vi "myPICO_ResultFFT.vi"(4 "是否需要第二台":bool, 5 "MultiBuffers 2":T1(array[cluster]), 6 "示波器量程":u16, 7 "MultiBuffers 1":T1(array[cluster]), 9 "Max Adc value 2":i16, 10 "Max Adc value":i16) -> (2 "数组":cdb[][](array[numeric]))   [LabVIEW 2024]
doc: "由于它的实际功能被合并进了myFFT_RowSave.vi\n（因为同步系模式需要在FFT前时域变换），\n实际上它并没有被在主程序中使用。"
uses:
  <vilib>/Analysis/2dsp.llb/Real FFT.vi
  <vilib>/Analysis/NI_AALPro.lvlib
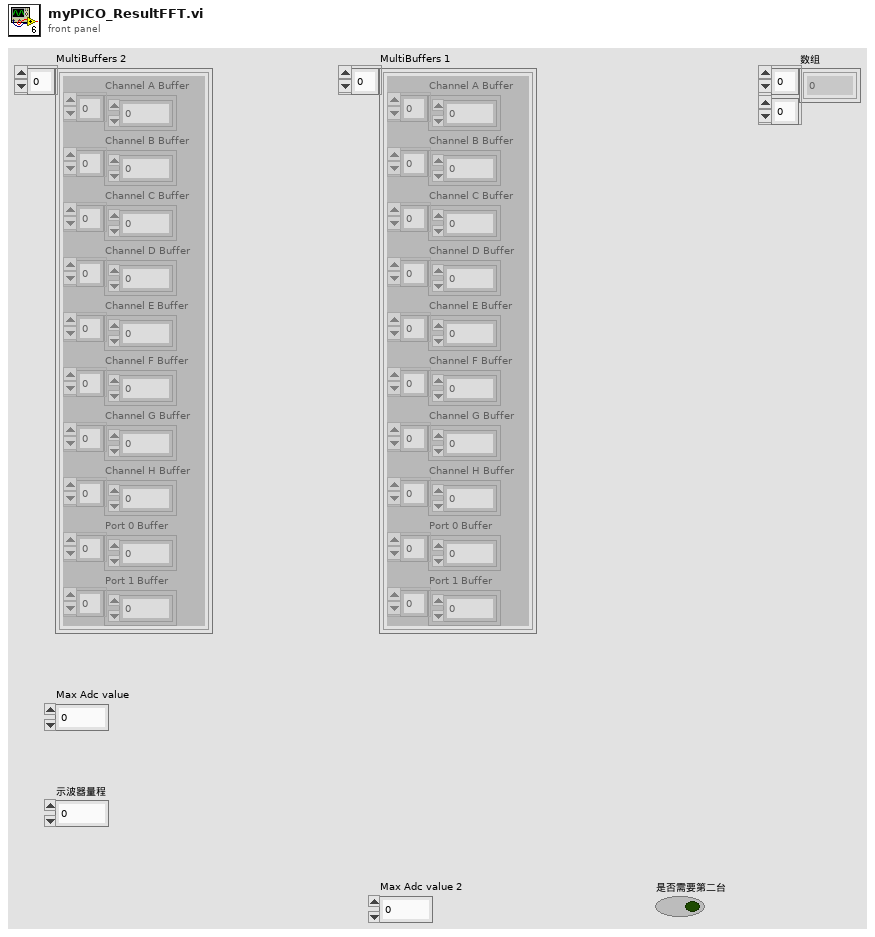
[diagram p1: front panel]
types:
  T1 = cluster{"Channel A Buffer":i16[], "Channel B Buffer":i16[], "Channel C Buffer":i16[], "Channel D Buffer":i16[], "Channel E Buffer":i16[], "Channel F Buffer":i16[], "Channel G Buffer":i16[], "Channel H Buffer":i16[], "Port 0 Buffer":i16[], "Port 1 Buffer":i16[]}[]
  T2 = cluster{"Channel A Buffer":i16[], "Channel B Buffer":i16[], "Channel C Buffer":i16[], "Channel D Buffer":i16[], "Channel E Buffer":i16[], "Channel F Buffer":i16[], "Channel G Buffer":i16[], "Channel H Buffer":i16[], "Port 0 Buffer":i16[], "Port 1 Buffer":i16[]}
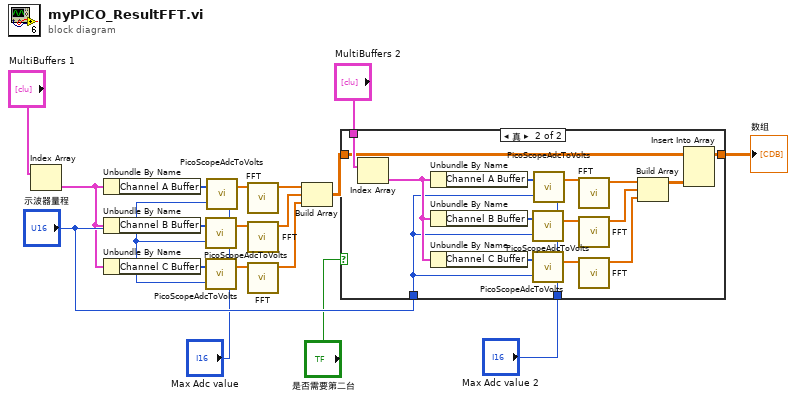
[diagram p0: block diagram]
diagram:
  n1 = Index Array(array="MultiBuffers 1") -> (element=w9:T2)  [unwired: 1 in]
  n2 = Unbundle By Name(w9) -> ("Channel A Buffer"=w7:i16[])
  n3 = Unbundle By Name(w9) -> ("Channel B Buffer"=w8:i16[])
  n4 = Unbundle By Name(w9) -> ("Channel C Buffer"=w6:i16[])
  n5 = call "PicoScopeAdcToVolts.vi"("Max_adc"="Max Adc value", "Range Index"="示波器量程", "Data"=w8) -> ("Data"=w4:dbl[])
  n6 = call "PicoScopeAdcToVolts.vi"("Max_adc"="Max Adc value", "Range Index"="示波器量程", "Data"=w6) -> ("Data"=w3:dbl[])
  n7 = call "PicoScopeAdcToVolts.vi"("Max_adc"="Max Adc value", "Range Index"="示波器量程", "Data"=w7) -> ("Data"=w5:dbl[])
  n8 = call-poly <vilib>:"FFT.vi"("X"=w5) -> ("FFT {X}"=w12:cdb[])  [unwired: 9 in, 1 out]
  n9 = call-poly <vilib>:"FFT.vi"("X"=w4) -> ("FFT {X}"=w13:cdb[])  [unwired: 9 in, 1 out]
  n10 = call-poly <vilib>:"FFT.vi"("X"=w3) -> ("FFT {X}"=w14:cdb[])  [unwired: 9 in, 1 out]
  n11 = Build Array(w12, w13, w14) -> (w15:cdb[][])
  n12 = case shown="真" "是否需要第二台" {
    tunnel: "MultiBuffers 2" -> [_ w28]
    tunnel: "Max Adc value 2" -> [_ w27]
    tunnel: w15 -> [w19 w23]
    tunnel: [w19 w21] -> w17
    tunnel: "示波器量程" -> [_ w20]
    frame False {
    }
    frame True {
      n13 = Index Array(array=w28) -> (element=w32:T2)  [unwired: 1 in]
      n14 = Unbundle By Name(w32) -> ("Channel A Buffer"=w30:i16[])
      n15 = Unbundle By Name(w32) -> ("Channel B Buffer"=w31:i16[])
      n16 = Unbundle By Name(w32) -> ("Channel C Buffer"=w29:i16[])
      n17 = call "PicoScopeAdcToVolts.vi"("Max_adc"=w27, "Range Index"=w20, "Data"=w31) -> ("Data"=w34:dbl[])
      n18 = call "PicoScopeAdcToVolts.vi"("Max_adc"=w27, "Range Index"=w20, "Data"=w29) -> ("Data"=w35:dbl[])
      n19 = call "PicoScopeAdcToVolts.vi"("Max_adc"=w27, "Range Index"=w20, "Data"=w30) -> ("Data"=w33:dbl[])
      n20 = call-poly <vilib>:"FFT.vi"("X"=w33) -> ("FFT {X}"=w26:cdb[])  [unwired: 9 in, 1 out]
      n21 = call-poly <vilib>:"FFT.vi"("X"=w34) -> ("FFT {X}"=w25:cdb[])  [unwired: 9 in, 1 out]
      n22 = call-poly <vilib>:"FFT.vi"("X"=w35) -> ("FFT {X}"=w24:cdb[])  [unwired: 9 in, 1 out]
      n23 = Build Array(w26, w25, w24) -> (w22:cdb[][])
      n24 = Insert Into Array(array=w23, new element=w22) -> (w21:cdb[][])  [unwired: 2 in]
    }
  }
  "数组" <- w17
